vi "HighCDischargeTime.vi"() -> ()   [LabVIEW 2020]
uses:
  <instrlib>/NH Research Regenerative Test Series/Public/Configure/Output Safety.ctl
  <vilib>/DAQmx/read.llb/DAQmx Read (Analog 1D DBL NChan 1Samp).vi
  <instrlib>/NH Research Regenerative Test Series/Public/Data/Read (Ave Current).vi
  <instrlib>/NH Research Regenerative Test Series/Public/Data/Low Level/Fetch (Ave Voltage).vi
  <instrlib>/NH Research Regenerative Test Series/Public/Data/Low Level/Fetch (Ave True Power).vi
  <vilib>/DAQmx/miscellaneous.llb/DAQmx Fill In Error Info.vi
  <instrlib>/NH Research Regenerative Test Series/NH Research Regenerative Test Series.lvlib
panel:
  in  "Wait time":dbl
  out "WaitElapsed Time (s)":dbl caption="Elapsed Time (s)"
  out "String 3":string
  out "Ave True Power (W) 3":dbl
  out "Ave Voltage (V) 3":dbl
  out "Ave Current (A) 3":dbl
  in  "Logical Instrument Number 3":u32=1
  in  "VISA resource name 3":refnum<visa-resource-name>
  out "String 2":string
  out "Ave True Power (W) 2":dbl
  out "Ave Voltage (V) 2":dbl
  out "Ave Current (A) 2":dbl
  in  "Logical Instrument Number 2":u32=1
  in  "VISA resource name 2":refnum<visa-resource-name>
  out "Temp2":dbl
  out "Temp1":dbl
  out "Task error out":errorcluster
  out "String":string
  in  "Output Safety":T1
  out "Filename Out":path
  in  "DAQmx Task Name":refnum<k21>
  in  "Path":path
  out "Ave Current (A)":dbl
  out "Ave Voltage (V)":dbl
  out "Ave True Power (W)":dbl
  out "Status Byte Register":T2
  in  "Logical Instrument Number":u32=1
  in  "Current Setpoint (0 A)":dbl format="%#.6g"
  in  "Battery Detect Voltage (0V)":dbl format="%#.6g"
  in  "VISA resource name":refnum<visa-resource-name>
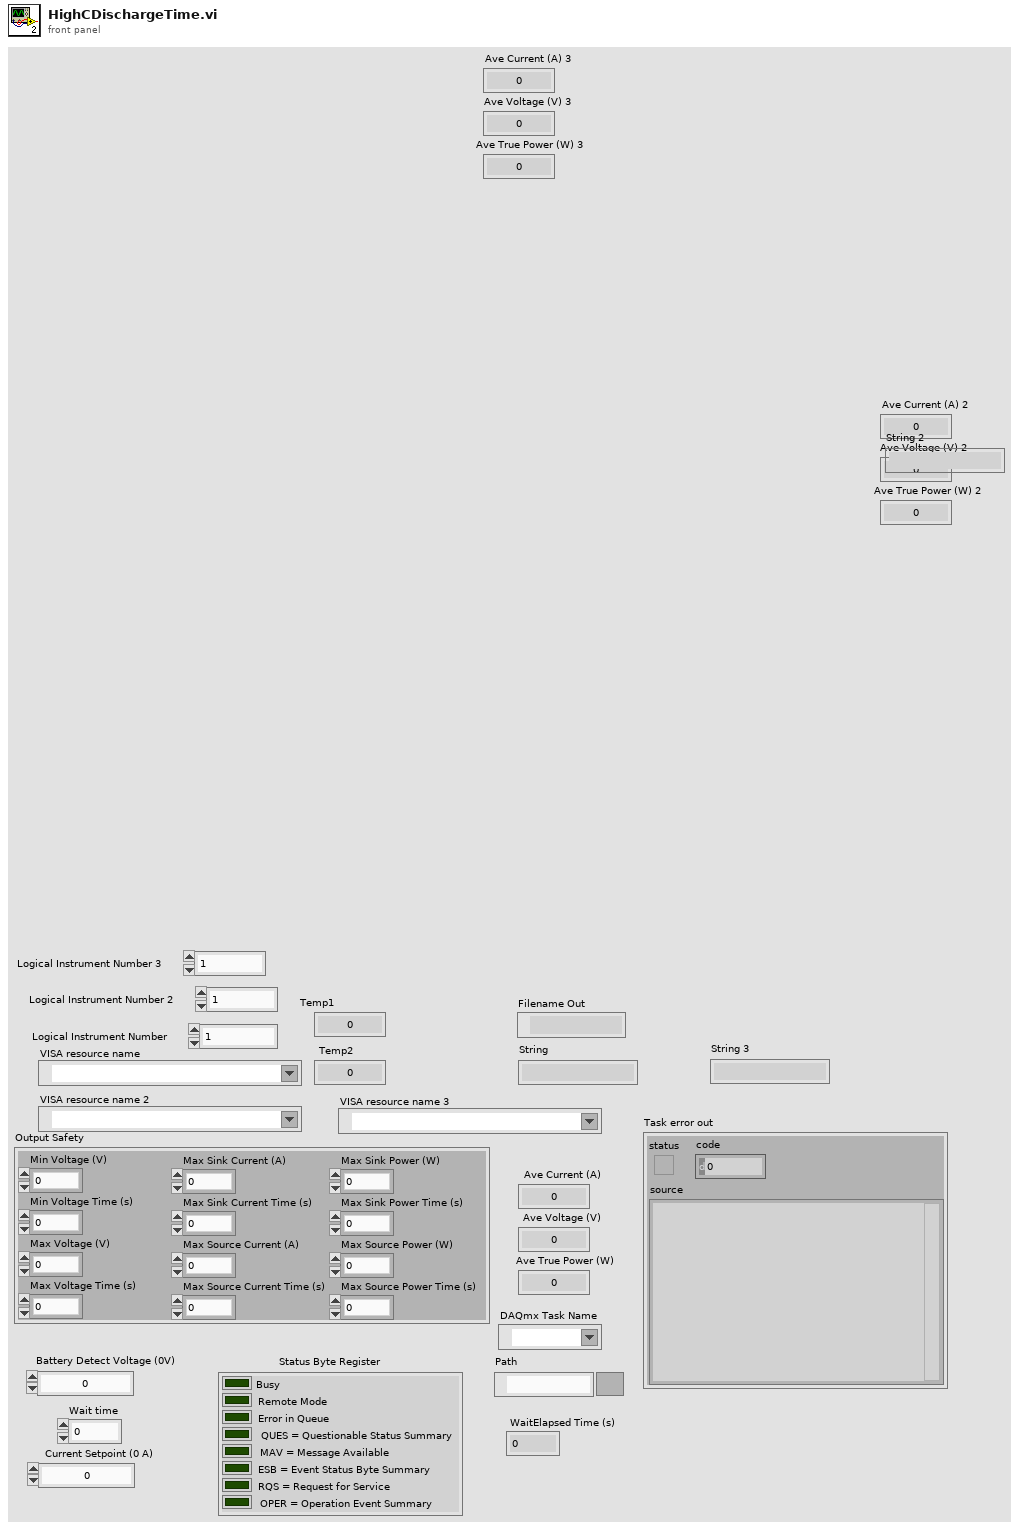
[diagram p1: front panel]
types:
  T1 = typedef "NH Research Regenerative Test Series.lvlib/Output Safety.ctl" = cluster{"Min Voltage (V)":dbl, "Min Voltage Time (s)":dbl, "Max Voltage (V)":dbl, "Max Voltage Time (s)":dbl, "Max Sink Current (A)":dbl, "Max Sink Current Time (s)":dbl, "Max Source Current (A)":dbl, "Max Source Current Time (s)":dbl, "Max Sink Power (W)":dbl, "Max Sink Power Time (s)":dbl, "Max Source Power (W)":dbl, "Max Source Power Time (s)":dbl}
  T2 = cluster{"Busy":bool, "Remote Mode":bool, "Error in Queue":bool, "QUES = Questionable Status Summary":bool, "MAV = Message Available":bool, "ESB = Event Status Byte Summary":bool, "RQS = Request for Service":bool, "OPER = Operation Event Summary":bool}
  T3 = cluster{"data[0]":dbl, "data[1]":dbl, "data[2]":dbl, "data[3]":dbl, "data[4]":dbl, "data[5]":dbl, "data[6]":dbl, "data[7]":dbl, "data[8]":dbl}
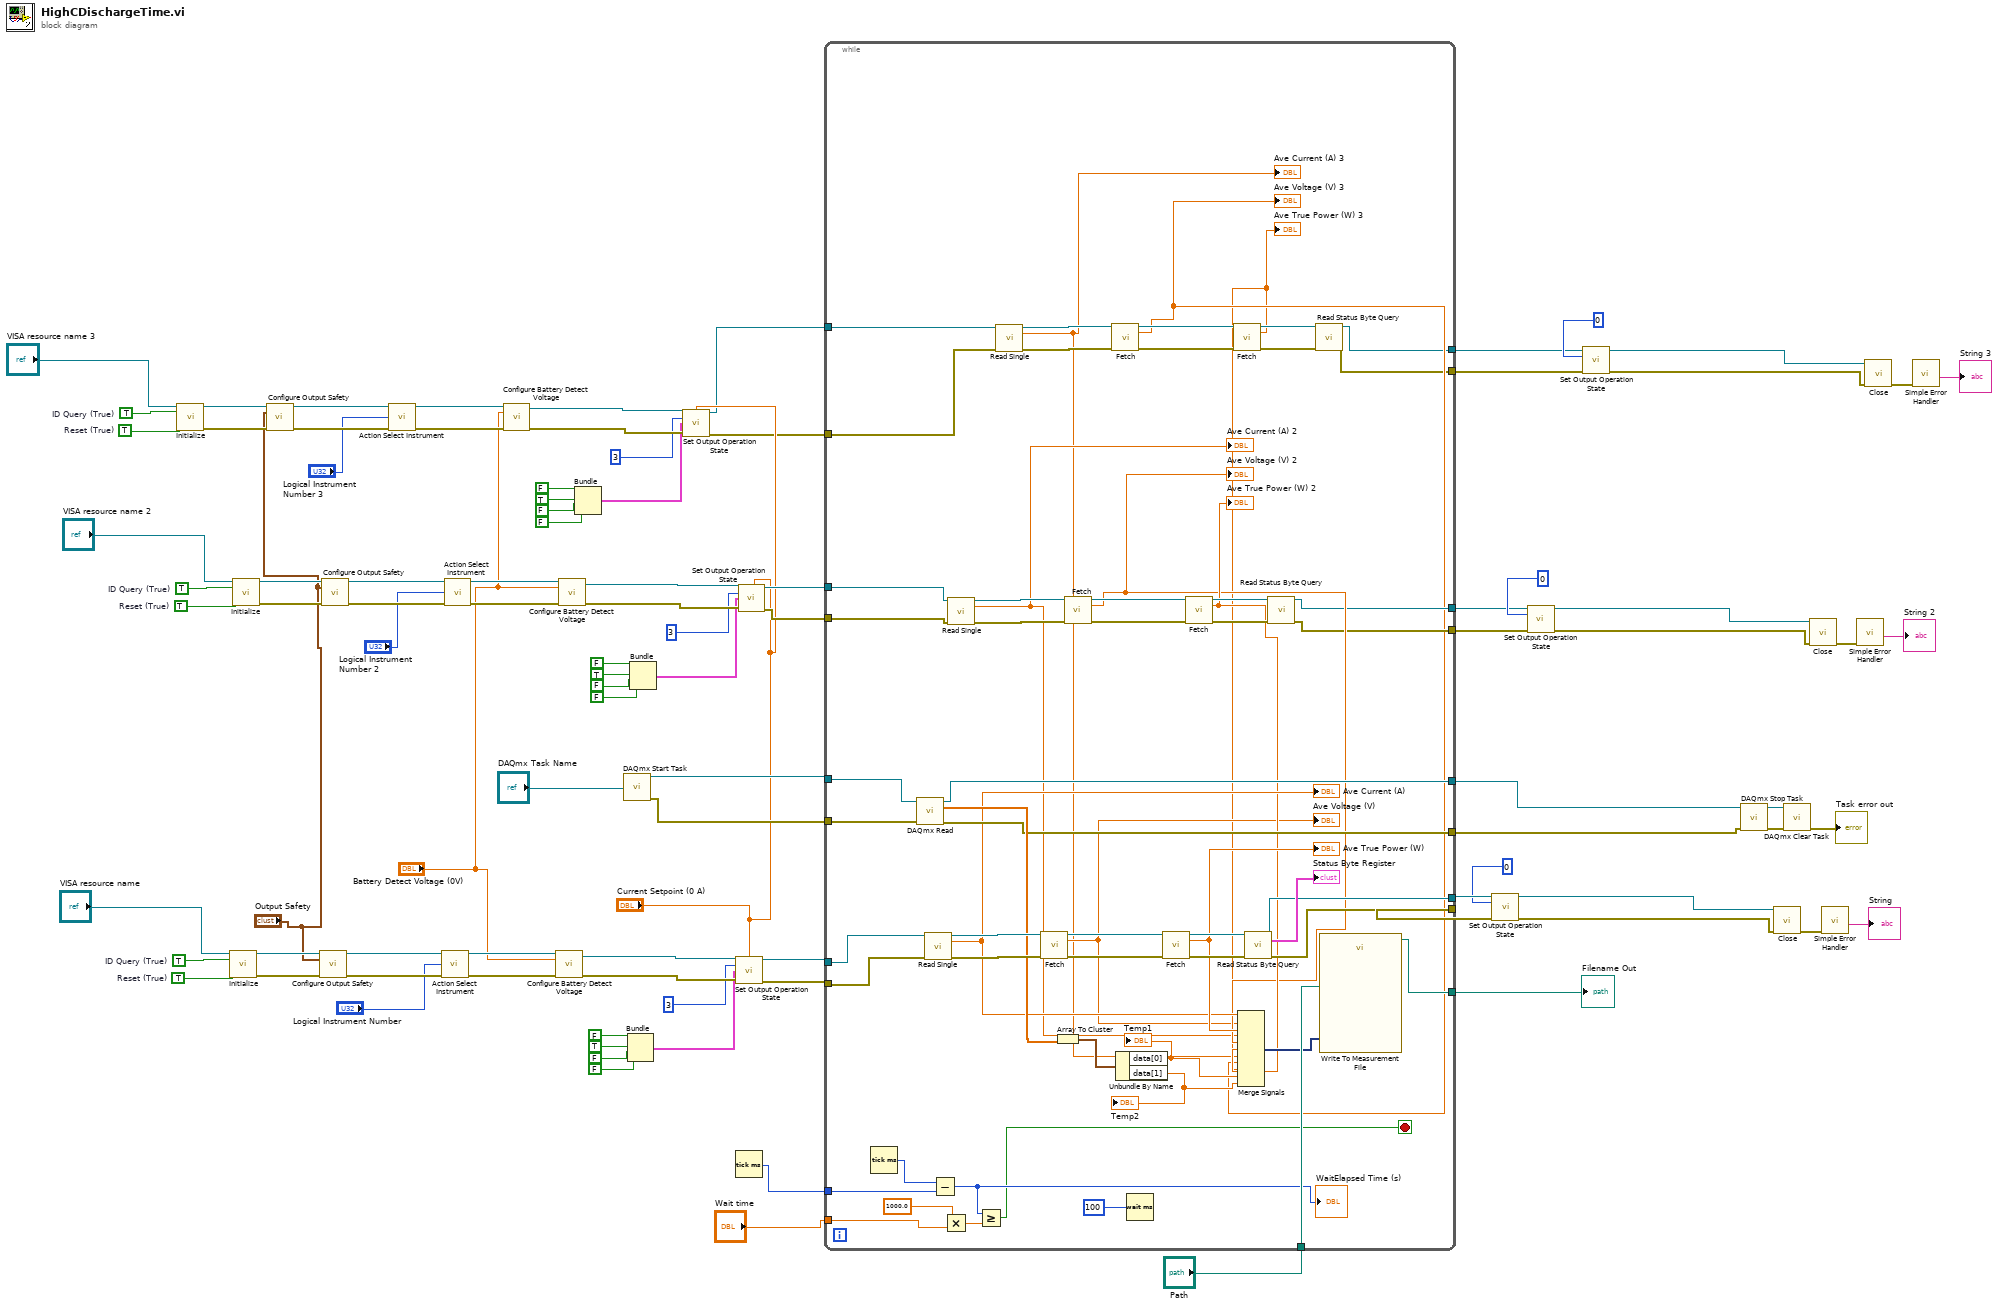
[diagram p0: block diagram]
diagram:
  w22 = TRUE  # ID Query (True)
  w21 = TRUE  # Reset (True)
  w50 = TRUE  # ID Query (True)
  w49 = TRUE  # Reset (True)
  w79 = TRUE  # ID Query (True)
  w78 = TRUE  # Reset (True)
  n1 = call <vilib>:"Initialize.vi"("VISA resource name"="VISA resource name 3", "ID Query (True)"=w22, "Reset (True)"=w21) -> ("VISA resource name out"=w20:refnum<visa-resource-name>, "error out"=w19:errorcluster)  [unwired: 11 in]
  n2 = call <vilib>:"Initialize.vi"("VISA resource name"="VISA resource name", "ID Query (True)"=w79, "Reset (True)"=w78) -> ("VISA resource name out"=w77:refnum<visa-resource-name>, "error out"=w76:errorcluster)  [unwired: 11 in]
  n3 = call <vilib>:"Initialize.vi"("VISA resource name"="VISA resource name 2", "ID Query (True)"=w50, "Reset (True)"=w49) -> ("VISA resource name out"=w48:refnum<visa-resource-name>, "error out"=w47:errorcluster)  [unwired: 11 in]
  n4 = call <vilib>:"Configure Output Safety.vi"("VISA resource name"=w20, "Output Safety"="Output Safety", "error in (no error)"=w19) -> ("VISA resource name out"=w17:refnum<visa-resource-name>, "error out"=w16:errorcluster)  [unwired: 11 in]
  n5 = call <vilib>:"Configure Output Safety.vi"("VISA resource name"=w77, "Output Safety"="Output Safety", "error in (no error)"=w76) -> ("VISA resource name out"=w74:refnum<visa-resource-name>, "error out"=w61:errorcluster)  [unwired: 11 in]
  n6 = call <vilib>:"Configure Output Safety.vi"("VISA resource name"=w48, "Output Safety"="Output Safety", "error in (no error)"=w47) -> ("VISA resource name out"=w45:refnum<visa-resource-name>, "error out"=w44:errorcluster)  [unwired: 11 in]
  n7 = call <instrlib>:"Action Select Instrument.vi"("VISA resource name"=w17, "Logical Instrument Number"="Logical Instrument Number 3", "error in (no error)"=w16) -> ("VISA resource name out"=w32:refnum<visa-resource-name>, "error out"=w31:errorcluster)  [unwired: 11 in]
  n8 = call <instrlib>:"Action Select Instrument.vi"("VISA resource name"=w74, "Logical Instrument Number"="Logical Instrument Number", "error in (no error)"=w61) -> ("VISA resource name out"=w96:refnum<visa-resource-name>, "error out"=w95:errorcluster)  [unwired: 11 in]
  n9 = call <instrlib>:"Action Select Instrument.vi"("VISA resource name"=w45, "Logical Instrument Number"="Logical Instrument Number 2", "error in (no error)"=w44) -> ("VISA resource name out"=w60:refnum<visa-resource-name>, "error out"=w59:errorcluster)  [unwired: 11 in]
  n10 = call <vilib>:"Configure Battery Detect Voltage.vi"("VISA resource name"=w32, "Battery Detect Voltage (0V)"="Battery Detect Voltage (0V)", "error in (no error)"=w31) -> ("VISA resource name out"=w30:refnum<visa-resource-name>, "error out"=w29:errorcluster)  [unwired: 11 in]
  n11 = call <vilib>:"Configure Battery Detect Voltage.vi"("VISA resource name"=w96, "Battery Detect Voltage (0V)"="Battery Detect Voltage (0V)", "error in (no error)"=w95) -> ("VISA resource name out"=w94:refnum<visa-resource-name>, "error out"=w93:errorcluster)  [unwired: 11 in]
  n12 = call <vilib>:"Configure Battery Detect Voltage.vi"("VISA resource name"=w60, "Battery Detect Voltage (0V)"="Battery Detect Voltage (0V)", "error in (no error)"=w59) -> ("VISA resource name out"=w58:refnum<visa-resource-name>, "error out"=w57:errorcluster)  [unwired: 11 in]
  n13 = Bundle(FALSE, TRUE, FALSE, FALSE) -> (w23:cluster{bool, bool, bool, bool})  [unwired: 1 in]
  n14 = call <vilib>:"DAQmx Start Task.vi"("task/channels in"="DAQmx Task Name") -> ("task out"=w72:refnum<k21>, "error out"=w62:errorcluster)  [unwired: 13 in]
  n15 = Bundle(FALSE, TRUE, FALSE, FALSE) -> (w82:cluster{bool, bool, bool, bool})  [unwired: 1 in]
  n16 = Bundle(FALSE, TRUE, FALSE, FALSE) -> (w51:cluster{bool, bool, bool, bool})  [unwired: 1 in]
  n17 = call <vilib>:"Set Output Operation State.vi"("VISA resource name"=w30, "Current Setpoint (0 A)"="Current Setpoint (0 A)", "Mode (0: Off)"=3, "Enable"=w23, "error in (no error)"=w29) -> ("VISA resource name out"=w11:refnum<visa-resource-name>, "error out"=w10:errorcluster)  [unwired: 9 in]
  n18 = call <vilib>:"Set Output Operation State.vi"("VISA resource name"=w94, "Current Setpoint (0 A)"="Current Setpoint (0 A)", "Mode (0: Off)"=3, "Enable"=w82, "error in (no error)"=w93) -> ("VISA resource name out"=w89:refnum<visa-resource-name>, "error out"=w88:errorcluster)  [unwired: 9 in]
  n19 = Tick Count (ms)() -> (millisecond timer value=w2:u32)
  n20 = call <vilib>:"Set Output Operation State.vi"("VISA resource name"=w58, "Current Setpoint (0 A)"="Current Setpoint (0 A)", "Mode (0: Off)"=3, "Enable"=w51, "error in (no error)"=w57) -> ("VISA resource name out"=w41:refnum<visa-resource-name>, "error out"=w40:errorcluster)  [unwired: 9 in]
  n21 = while {
    tunnel: w89 -> [w149]
    tunnel: w88 -> [w148]
    tunnel: [w146] -> w92
    tunnel: [w145] -> w91
    tunnel: "Path" -> [w143]
    tunnel: w72 -> [w142]
    tunnel: [w138] -> w64
    tunnel: [w137] -> w63
    tunnel: w62 -> [w136]
    tunnel: [w135] -> w80
    tunnel: w41 -> [w123]
    tunnel: w40 -> [w122]
    tunnel: [w121] -> w34
    tunnel: [w120] -> w33
    tunnel: w11 -> [w112]
    tunnel: w10 -> [w111]
    tunnel: [w105] -> w4
    tunnel: [w104] -> w3
    tunnel: w2 -> [w99]
    tunnel: "Wait time" -> [w98]
    stop <- w97 stop-if-true
    n22 = Tick Count (ms)() -> (millisecond timer value=w103:u32)
    n23 = call-poly <vilib>:"DAQmx Read.vi"("task/channels in"=w142, "error in"=w136) -> ("task out"=w138:refnum<k21>, "data"=w141:dbl[], "error out"=w137:errorcluster)  [unwired: 11 in]
    n24 = call-poly <instrlib>:"Read Single.vi"("VISA resource name"=w149, "error in (no error)"=w148) -> ("VISA resource name out"=w154:refnum<visa-resource-name>, "Ave Current (A)"=w134:dbl, "error out"=w155:errorcluster)  [unwired: 11 in]
    "Ave Current (A)" <- w134
    n25 = Subtract(x=w103, y=w99) -> (x-y=w102:u32)
    "WaitElapsed Time (s)" <- w102
    n26 = Multiply(x=1000.0, y=w98) -> (x*y=w101:dbl)
    n27 = call-poly <instrlib>:"Read Single.vi"("VISA resource name"=w123, "error in (no error)"=w122) -> ("VISA resource name out"=w131:refnum<visa-resource-name>, "Ave Current (A)"=w124:dbl, "error out"=w132:errorcluster)  [unwired: 11 in]
    "Ave Current (A) 2" <- w124
    n28 = Greater Or Equal?(x=w102, y=w101) -> (x >= y?=w97:bool)
    n29 = call-poly <instrlib>:"Read Single.vi"("VISA resource name"=w112, "error in (no error)"=w111) -> ("VISA resource name out"=w117:refnum<visa-resource-name>, "Ave Current (A)"=w108:dbl, "error out"=w118:errorcluster)  [unwired: 11 in]
    "Ave Current (A) 3" <- w108
    n30 = call-poly <instrlib>:"Fetch.vi"("VISA resource name"=w154, "error in (no error)"=w155) -> ("VISA resource name out"=w153:refnum<visa-resource-name>, "Ave Voltage (V)"=w119:dbl, "error out"=w152:errorcluster)  [unwired: 11 in]
    "Ave Voltage (V)" <- w119
    n31 = Array To Cluster(array=w141) -> (cluster=w140:T3)
    n32 = call-poly <instrlib>:"Fetch.vi"("VISA resource name"=w131, "error in (no error)"=w132) -> ("VISA resource name out"=w130:refnum<visa-resource-name>, "Ave Voltage (V)"=w125:dbl, "error out"=w129:errorcluster)  [unwired: 11 in]
    "Ave Voltage (V) 2" <- w125
    n33 = call-poly <instrlib>:"Fetch.vi"("VISA resource name"=w117, "error in (no error)"=w118) -> ("VISA resource name out"=w116:refnum<visa-resource-name>, "Ave Voltage (V)"=w107:dbl, "error out"=w115:errorcluster)  [unwired: 11 in]
    "Ave Voltage (V) 3" <- w107
    n34 = Unbundle By Name(w140) -> ("data[0]"=w110:dbl, "data[1]"=w109:dbl)
    "Temp1" <- w110
    "Temp2" <- w109
    n35 = Wait (ms)(milliseconds to wait=100) -> ()  [unwired: 1 out]
    n36 = call-poly <instrlib>:"Fetch.vi"("VISA resource name"=w153, "error in (no error)"=w152) -> ("VISA resource name out"=w151:refnum<visa-resource-name>, "Ave True Power (W)"=w144:dbl, "error out"=w150:errorcluster)  [unwired: 11 in]
    "Ave True Power (W)" <- w144
    n37 = call-poly <instrlib>:"Fetch.vi"("VISA resource name"=w130, "error in (no error)"=w129) -> ("VISA resource name out"=w128:refnum<visa-resource-name>, "Ave True Power (W)"=w126:dbl, "error out"=w127:errorcluster)  [unwired: 11 in]
    "Ave True Power (W) 2" <- w126
    n38 = call-poly <instrlib>:"Fetch.vi"("VISA resource name"=w116, "error in (no error)"=w115) -> ("VISA resource name out"=w114:refnum<visa-resource-name>, "Ave True Power (W)"=w106:dbl, "error out"=w113:errorcluster)  [unwired: 11 in]
    "Ave True Power (W) 3" <- w106
    n39 = Merge Signals "Merge Signals"(w134, w119, w144, w124, w125, w126, w108, w107, w106, w110, w109) -> (w139:dynamicdata)
    n40 = call <instrlib>:"Read Status Byte Query.vi"("VISA resource name"=w151, "error in (no error)"=w150) -> ("VISA resource name out"=w146:refnum<visa-resource-name>, "Status Byte Register"=→"Status Byte Register":T2, "error out"=w145:errorcluster)  [unwired: 11 in]
    n41 = call <instrlib>:"Read Status Byte Query.vi"("VISA resource name"=w128, "error in (no error)"=w127) -> ("VISA resource name out"=w121:refnum<visa-resource-name>, "error out"=w120:errorcluster)  [unwired: 11 in, 1 out]
    n42 = call <instrlib>:"Read Status Byte Query.vi"("VISA resource name"=w114, "error in (no error)"=w113) -> ("VISA resource name out"=w105:refnum<visa-resource-name>, "error out"=w104:errorcluster)  [unwired: 11 in, 1 out]
    n43 = call "Write To Measurement File"("Signals"=w139, "Filename"=w143) -> ("Filename Out"=w135:path)  [unwired: 15 in, 2 out]
  }
  "Filename Out" <- w80
  n44 = call <vilib>:"Set Output Operation State.vi"("VISA resource name"=w92, "Mode (0: Off)"=0, "error in (no error)"=w91) -> ("VISA resource name out"=w66:refnum<visa-resource-name>, "error out"=w65:errorcluster)  [unwired: 11 in]
  n45 = call <vilib>:"Set Output Operation State.vi"("VISA resource name"=w34, "Mode (0: Off)"=0, "error in (no error)"=w33) -> ("VISA resource name out"=w36:refnum<visa-resource-name>, "error out"=w35:errorcluster)  [unwired: 11 in]
  n46 = call <vilib>:"Set Output Operation State.vi"("VISA resource name"=w4, "Mode (0: Off)"=0, "error in (no error)"=w3) -> ("VISA resource name out"=w6:refnum<visa-resource-name>, "error out"=w5:errorcluster)  [unwired: 11 in]
  n47 = call <vilib>:"DAQmx Stop Task.vi"("task/channels in"=w64, "error in"=w63) -> ("task out"=w70:refnum<k21>, "error out"=w69:errorcluster)  [unwired: 12 in]
  n48 = call <instrlib>:"Close.vi"("VISA resource name"=w66, "error in (no error)"=w65) -> ("error out"=w67:errorcluster)  [unwired: 13 in]
  n49 = call <vilib>:"DAQmx Clear Task.vi"("task in"=w70, "error in"=w69) -> ("error out"=→"Task error out":errorcluster)  [unwired: 13 in]
  n50 = call <instrlib>:"Close.vi"("VISA resource name"=w36, "error in (no error)"=w35) -> ("error out"=w37:errorcluster)  [unwired: 13 in]
  n51 = call <vilib>:"Simple Error Handler.vi"("error in (no error)"=w67) -> ("source out"=→"String":string)  [unwired: 4 in, 4 out]
  n52 = call <vilib>:"Simple Error Handler.vi"("error in (no error)"=w37) -> ("source out"=→"String 2":string)  [unwired: 4 in, 4 out]
  n53 = call <instrlib>:"Close.vi"("VISA resource name"=w6, "error in (no error)"=w5) -> ("error out"=w7:errorcluster)  [unwired: 13 in]
  n54 = call <vilib>:"Simple Error Handler.vi"("error in (no error)"=w7) -> ("source out"=→"String 3":string)  [unwired: 4 in, 4 out]
